vi "FA_ConvertFromSharedVariables.vi"(8 "Error In":errorcluster, 11 "Shared Variable":T1) -> (0 "Error Out":errorcluster, 3 "Config":T2)   [LabVIEW 2013, in "FA_SharedVariables.lvlib"]
doc: "Conferts from the Shared Variable typedef to a general config typedef"
uses:
  FA_SharedVariables.lvlib
  FA_NativeTypes API/source/VI Source/FA_Config.ctl
  FA_LocalStore API/source/VI Source/FA_LSSpecialTypes.ctl
  FA_SharedVariables.ctl
  FA_LocalStore API/source/VI Source/FA_LocalStore.lvlib
  FA_NativeTypes API/source/VI Source/FA_NativeTypes.lvlib
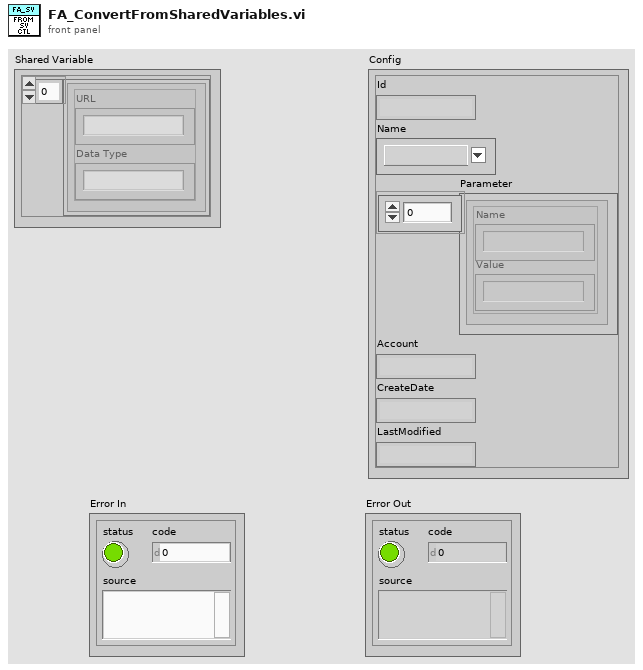
[diagram p1: front panel]
types:
  T1 = typedef "FA_SharedVariables.lvlib/FA_SharedVariables.ctl" = cluster{"Shared Variables":cluster{"URL":string, "Data Type":string}[]}
  T2 = typedef "FA_NativeTypes.lvlib/FA_Config.ctl" = cluster{"Id":string, "Name":T3, "Parameter":cluster{"Name":string, "Value":string}[], "Account":string, "CreateDate":string, "LastModified":string}
  T3 = typedef "FA_LocalStore.lvlib/FA_LSSpecialTypes.ctl" = string
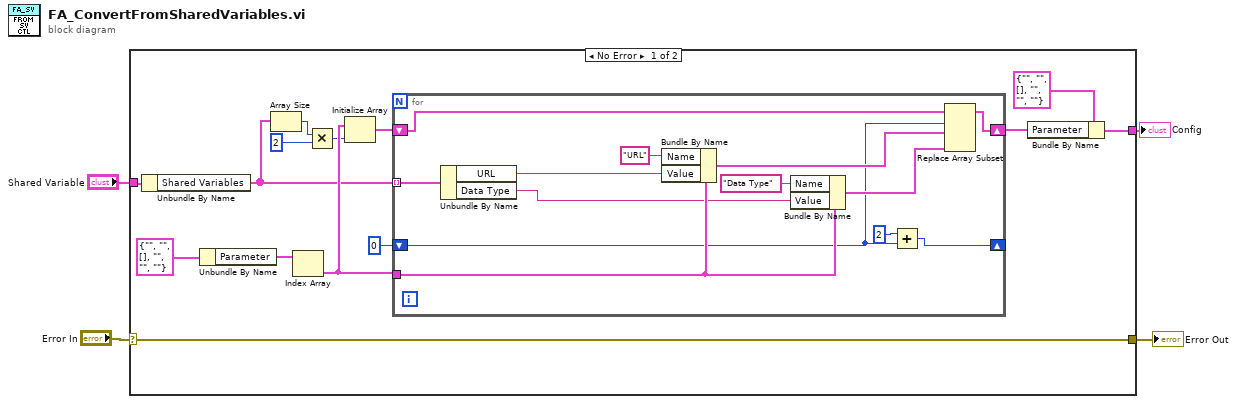
[diagram p0: block diagram]
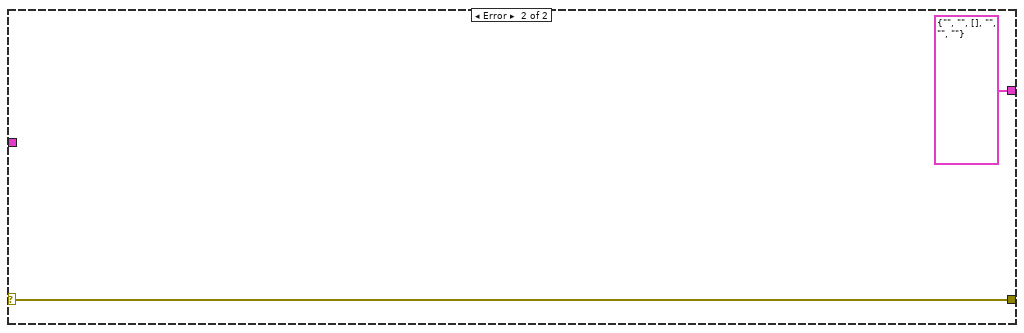
[diagram p2: hidden frame]
diagram:
  n1 = case shown="No Error" "Error In" {
    selector: "Error In" -> [w5 w32]
    tunnel: "Shared Variable" -> [w10 _]
    tunnel: [w6 T2 {"Id"="", "Name"="", "Parameter"=[], "Account"="", "CreateDate"="", "LastModified"=""} ("Config")] -> w3
    tunnel: [w5 w32] -> w1
    frame No Error {
      n2 = Unbundle By Name(w10) -> ("Shared Variables"=w9:cluster{"URL":string, "Data Type":string}[])
      n3 = Unbundle By Name(T2 {"Id"="", "Name"="", "Parameter"=[], "Account"="", "CreateDate"="", "LastModified"=""} ("Config")) -> ("Parameter"=w16:cluster{"Name":string, "Value":string}[])
      n4 = Array Size(array=w9) -> (size(s)=w18:i32)
      n5 = Index Array(array=w16) -> (element=w12:cluster{"Name":string, "Value":string})  [unwired: 1 in]
      n6 = Multiply(x=w18, y=2) -> (x*y=w8:i32)
      n7 = Initialize Array(w12, w8) -> (w11:cluster{"Name":string, "Value":string}[])
      n8 = for {
        tunnel: w12 -> [w25]
        shift-right: [w20] -> _
        shift-left: 0 ("index") -> [w21]
        shift-right: [w29] -> w13
        shift-left: w11 -> [w31]
        tunnel: w9 -> [w28] mode=indexing
        n9 = Unbundle By Name(w28) -> ("URL"=w27:string, "Data Type"=w24:string)
        n10 = Bundle By Name(cluster=w25, "Name"="URL", "Value"=w27) -> (w23:cluster{"Name":string, "Value":string})
        n11 = Bundle By Name(cluster=w25, "Name"="Data Type", "Value"=w24) -> (w22:cluster{"Name":string, "Value":string})
        n12 = Add(x=2, y=w21) -> (x+y=w20:i32)
        n13 = Replace Array Subset(array=w31, new element #1=w23, index #1=w21, new element #2=w22) -> (w29:cluster{"Name":string, "Value":string}[])  [unwired: 1 in]
      }
      n14 = Bundle By Name(cluster=T2 {"Id"="", "Name"="", "Parameter"=[], "Account"="", "CreateDate"="", "LastModified"=""} ("Config"), "Parameter"=w13) -> (w6:T2)
    }
    frame Error {
    }
  }
  "Config" <- w3
  "Error Out" <- w1
